vi "interface.vi"() -> ()   [LabVIEW 2022 SP3]
uses:
  <vilib>/Instr/_visa.llb/VISA Configure Serial Port (Instr).vi
panel:
  out "Current angle value":dbl
  out "Angle Chart":dbl(graph)
  out "Error":dbl(knob) scale=-25.0..25.0
  in  "START":bool
  out "Error Chart":dbl(graph)
  out "Error value":string
  in  "VISA resource name":refnum<visa-resource-name>
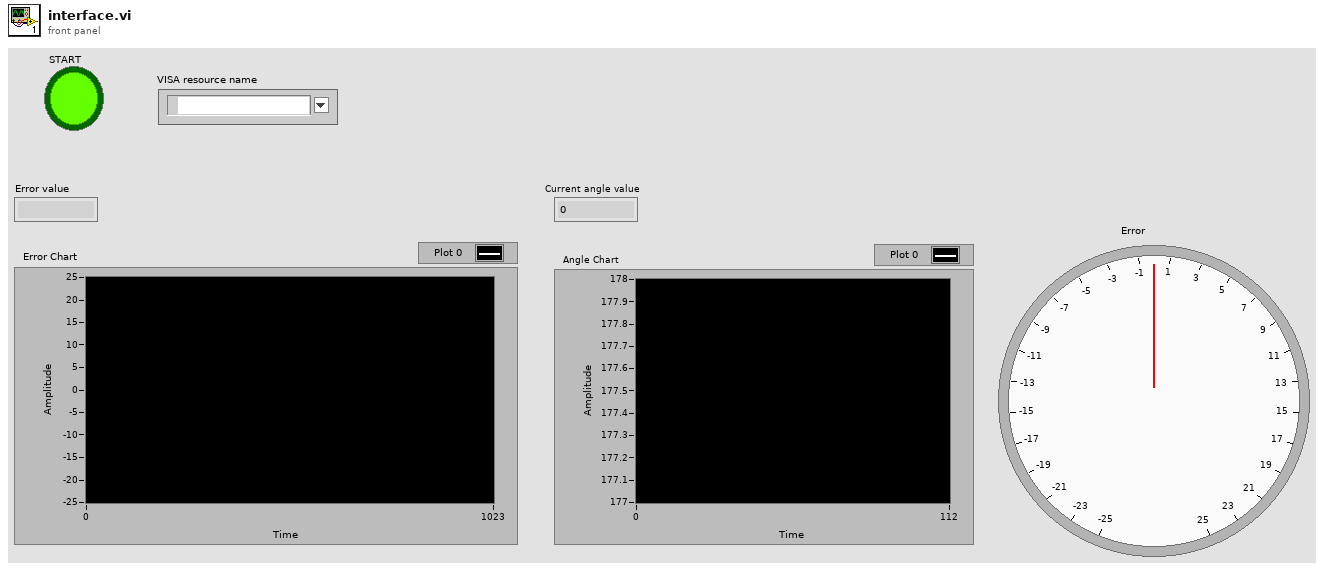
[diagram p1: front panel]
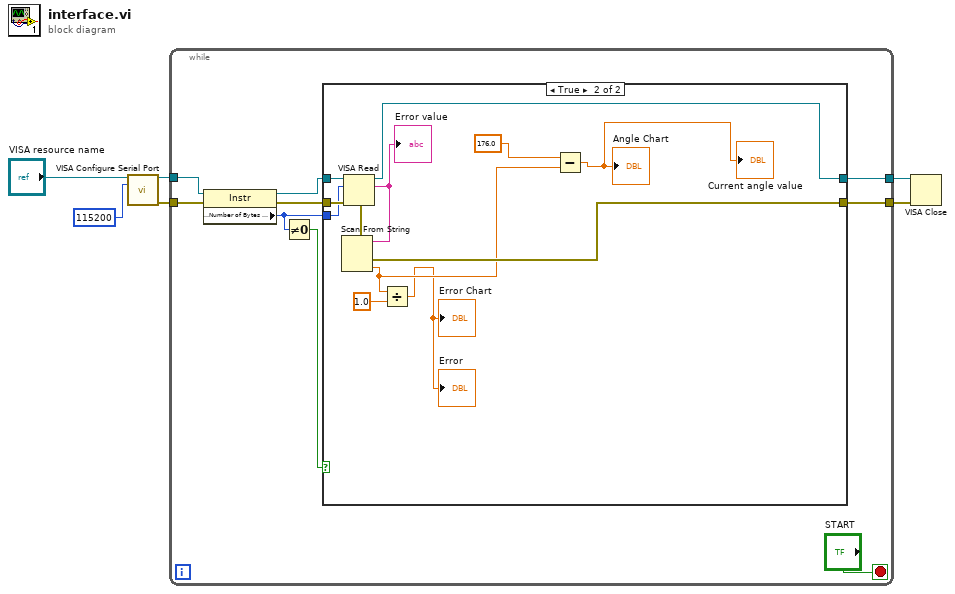
[diagram p0: block diagram]
diagram:
  n1 = call-poly "VISA Configure Serial Port"("VISA resource name"="VISA resource name", "baud rate (9600)"=u32 115200) -> ("VISA resource name out"=w5:refnum<visa-resource-name>, "error out"=w4:errorcluster)  [unwired: 12 in]
  n2 = while {
    tunnel: w5 -> [w14]
    tunnel: w4 -> [w15]
    tunnel: [w11] -> w2
    tunnel: [w10] -> w1
    stop <- "START" stop-if-true
    n3 = property class="Instr"(reference=w14, error in=w15) -> (reference out=w12:refnum<visa-resource-name>, error out=w13:errorcluster, "Serial Settings:Number of Bytes at Serial Port"=w8:u32)
    n4 = Not Equal To 0?(x=w8) -> (x != 0?=w9:bool)
    n5 = case shown="True" w9 {
      tunnel: w13 -> [w16 w29]
      tunnel: w12 -> [w17 w28]
      tunnel: w8 -> [_ w27]
      tunnel: [w17 w24] -> w11
      tunnel: [w16 w23] -> w10
      frame False {
      }
      frame True {
        n6 = VISA Read(VISA resource name=w28, byte count=w27, error in (no error)=w29) -> (VISA resource name out=w24:refnum<visa-resource-name>, read buffer=w26:string, error out=w25:errorcluster)  [unwired: 1 out]
        "Error value" <- w26
        n7 = Scan From String(input string=w26, error in=w25) -> (error out=w23:errorcluster, output 1=w20:dbl)  [unwired: 3 in, 2 out]
        n8 = Divide(x=w20, y=1.0) -> (x/y=→"Error Chart" →"Error":dbl)
        n9 = Subtract(x=176.0, y=w20) -> (x-y=→"Angle Chart" →"Current angle value":dbl)
      }
    }
  }
  n10 = VISA Close(VISA resource name=w2, error in (no error)=w1) -> ()  [unwired: 1 out]
